vi "控件大小读取.vi"(8 "错误输入（无错误）":errorcluster, 11 "控件引用输入":refnum<vi>) -> (0 "错误输出":errorcluster, 2 "边界":T1, 3 "引用输出":refnum<vi>)   [LabVIEW 8.6, in "窗口操作.lvlib"]
uses:
  <vilib>/Utility/miscctls.llb/LVBoundsTypeDef.ctl
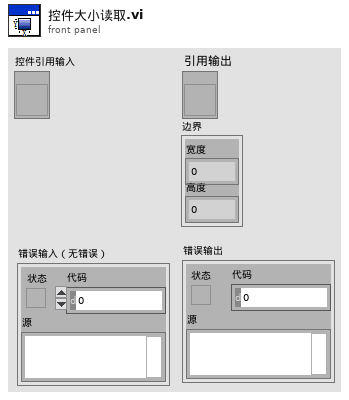
[diagram p1: front panel]
types:
  T1 = typedef "LVBoundsTypeDef.ctl" = cluster{"Width":u32, "Height":u32}
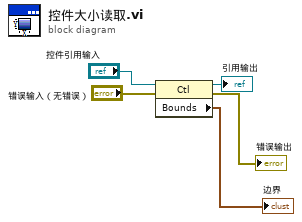
[diagram p0: block diagram]
diagram:
  n1 = property on="Property Node" class="Ctl"(reference="控件引用输入", error in="错误输入（无错误）") -> (reference out=→"引用输出":refnum<vi>, error out=→"错误输出":errorcluster, "Bounds"=→"边界":T1)
